vi "Recursive Folder List2.vi"(4 "Folders to Exclude\nREP ( ^[_.] as Default)\nempty to disable this feature":string="^[_.]", 6 "pattern":string, 8 "error in (no error)":errorcluster, 9 "Continue Recursing on Error? (F)":bool, 11 "Folder Path":path) -> (0 "error out":errorcluster, 1 "Number of Folders":i32, 2 "All Folders":path[](array[path]), 3 "dup Folder Path":path)   [LabVIEW 2017]
doc: "Recursively lists every folder under Folder Path whose name matches pattern. Folders to Exclude takes a regular expression and defaults to ^[_.], so hidden and underscore-prefixed folders are skipped."
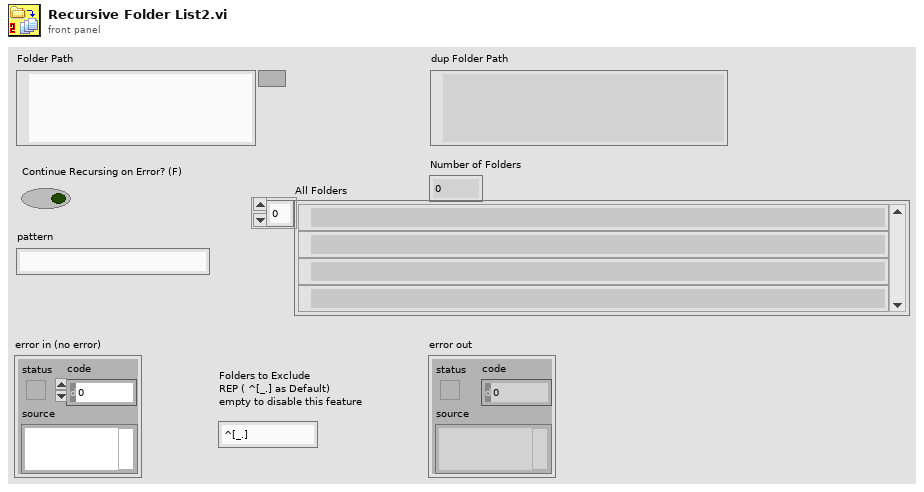
[diagram p1: front panel]
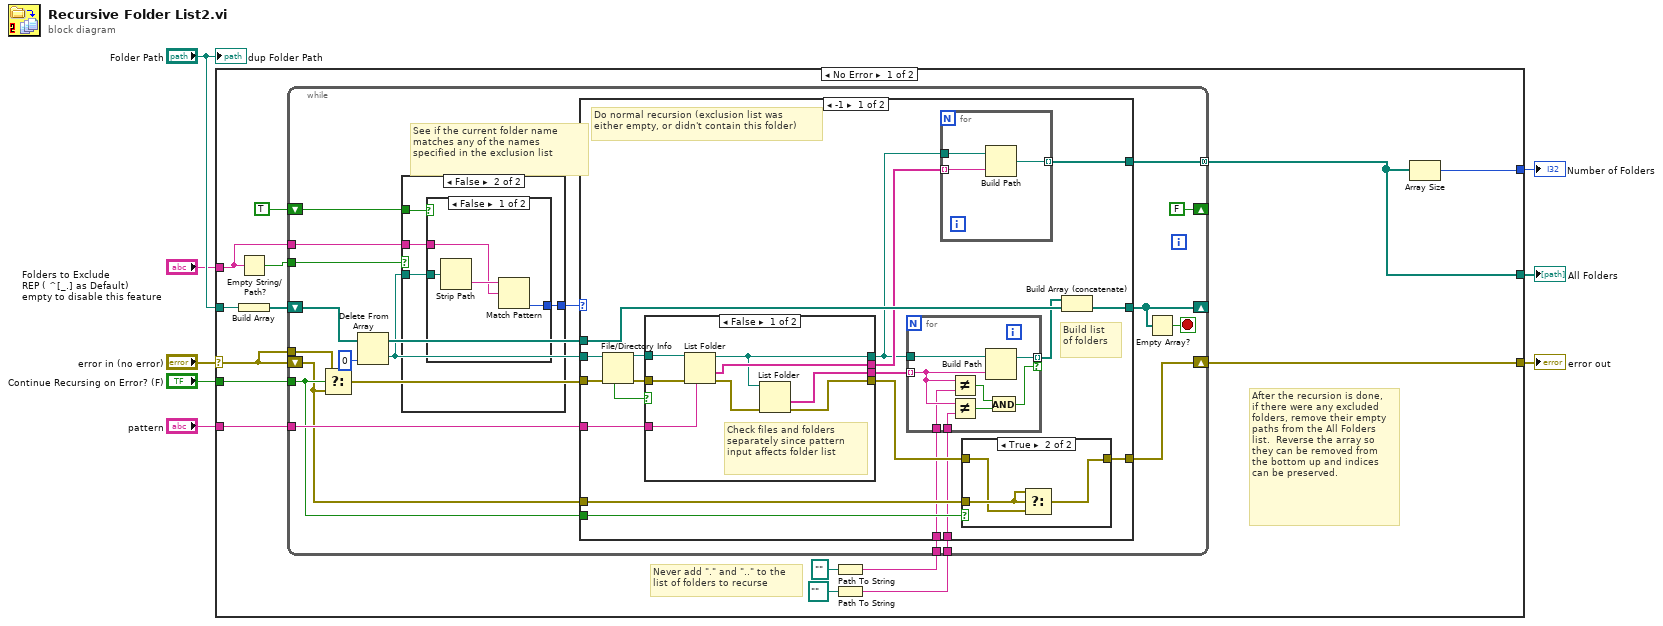
[diagram p0: block diagram]
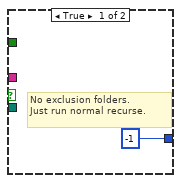
[diagram p2: hidden frame]
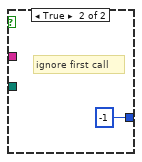
[diagram p3: hidden frame]
diagram:
  n1 = case shown="No Error" "error in (no error)" {
    selector: "error in (no error)" -> [w17 w100]
    tunnel: "Folder Path" -> [w23 _]
    tunnel: [w19 _] -> w8
    tunnel: [w20 w100] -> w7
    tunnel: [w9 _] -> w5
    tunnel: "pattern" -> [w21 _]
    tunnel: "Continue Recursing on Error? (F)" -> [w18 _]
    tunnel: "Folders to Exclude\nREP ( ^[_.] as Default)\nempty to disable this feature" -> [w11 _]
    frame No Error {
      # "Never add \".\" and \"..\" to the list of folders to recurse"
      # "After the recursion is done,\nif there were any excluded\nfolders, remove their empty\npaths from the All Folders\nlist.  Reverse the array so\nthey can be removed from\nthe bottom up and indices\ncan be preserved."
      n2 = Empty String/Path?(string/path=w11) -> (empty?=w12:bool)
      n3 = Build Array(w23) -> (w22:path[])
      n4 = Path To String(path=path "") -> (string=w14:string)
      n5 = Path To String(path=path "..") -> (string=w13:string)
      n6 = while {
        shift-left: w22 -> [w43]
        shift-right: [w41] -> _
        shift-right: [w35] -> w20
        shift-left: w17 -> [w34]
        tunnel: w21 -> [w42]
        tunnel: w18 -> [w36]
        tunnel: w17 -> [w37]
        tunnel: w11 -> [w31]
        tunnel: w12 -> [w32]
        tunnel: w14 -> [w28]
        tunnel: w13 -> [w27]
        shift-right: [FALSE] -> _
        shift-left: TRUE -> [w26]
        tunnel: [w24] -> w9 mode=concatenating
        stop <- w40 stop-if-true
        # "See if the current folder name\nmatches any of the names\nspecified in the exclusion list"
        n7 = Select(t=w37, s=w36, f=w34) -> (s? t:f=w38:errorcluster)
        n8 = Delete From Array(array=w43, index=0) -> (deleted portion=w30:path, array with subset deleted=w33:path[])  [unwired: 1 in]
        n9 = case shown="False" w32 {
          tunnel: w31 -> [_ w47]
          tunnel: w30 -> [_ w48]
          tunnel: [-1 ("index of element") w46] -> w29
          tunnel: w26 -> [_ w45]
          frame True {
            # "No exclusion folders.\nJust run normal recurse."
          }
          frame False {
            n10 = case shown="False" w45 {
              tunnel: w48 -> [w52 _]
              tunnel: w47 -> [w50 _]
              tunnel: [w49 -1 ("offset past match")] -> w46
              frame False {
                n11 = Strip Path(path=w52) -> (name=w51:string)  [unwired: 1 out]
                n12 = Match Pattern(string=w51, regular expression=w50) -> (offset past match=w49:i32)  [unwired: 1 in, 3 out]
              }
              frame True {
                # "ignore first call"
              }
            }
          }
        }
        n13 = case shown="-1" w29 {
          tunnel: w42 -> [w72 _]
          tunnel: [w70 w99] -> w41
          tunnel: w30 -> [w60 _]
          tunnel: w38 -> [w66 w98]
          tunnel: w36 -> [w64 _]
          tunnel: [w63 w98] -> w35
          tunnel: w34 -> [w62 _]
          tunnel: w33 -> [w61 w99]
          tunnel: w28 -> [w58 _]
          tunnel: w27 -> [w57 _]
          tunnel: [w54 _] -> w24
          frame -1 {
            # "Build list\nof folders"
            # "Do normal recursion (exclusion list was\neither empty, or didn't contain this folder)"
            n14 = File/Directory Info(path=w60, error in=w66) -> (path out=w68:path, error out=w69:errorcluster, shortcut=w67:bool)  [unwired: 4 out]
            n15 = case shown="False" w67 {
              tunnel: [w91 _] -> w56
              tunnel: [w90 w93] -> w55
              tunnel: [w89 w92] -> w65
              tunnel: w72 -> [w88 _]
              tunnel: [w84 _] -> w71
              tunnel: w69 -> [w87 w92]
              tunnel: w68 -> [w86 w93]
              frame False {
                # "Check files and folders\nseparately since pattern\ninput affects folder list"
                n16 = List Folder(path=w86, pattern=w88, error in=w87) -> (path out=w90:path, folder names=w91:string[], error out=w85:errorcluster)  [unwired: 2 out]
                n17 = List Folder(path=w90, error in=w85) -> (folder names=w84:string[], error out=w89:errorcluster)  [unwired: 4 out]
              }
              frame True {
                # "Do not attempt to recurse the contents of folder shortcuts"
              }
            }
            n18 = for {
              tunnel: w55 -> [w83]
              tunnel: [w82] -> w59 mode=indexing if=w81
              tunnel: w71 -> [w80] mode=indexing
              tunnel: w58 -> [w79]
              tunnel: w57 -> [w78]
              n19 = Not Equal?(x=w80, y=w79) -> (x != y?=w76:bool)
              n20 = Not Equal?(x=w80, y=w78) -> (x != y?=w77:bool)
              n21 = Build Path(base path=w83, name or relative path=w80) -> (appended path=w82:path)
              n22 = And(x=w76, y=w77) -> (x .and. y?=w81:bool)
            }
            n23 = for {
              tunnel: w56 -> [w75] mode=indexing
              tunnel: w55 -> [w74]
              tunnel: [w73] -> w54 mode=indexing
              n24 = Build Path(base path=w74, name or relative path=w75) -> (appended path=w73:path)
            }
            n25 = case shown="True" w64 {
              tunnel: w65 -> [w94 w96]
              tunnel: [w94 w95] -> w63
              tunnel: w62 -> [_ w97]
              frame False {
              }
              frame True {
                n26 = Select(t=w97, s=w97, f=w96) -> (s? t:f=w95:errorcluster)
              }
            }
            n27 = Build Array (concatenate)(w59, w61) -> (w70:path[])
          }
          frame Default {
            # "Output empty folder path here"
          }
        }
        n28 = Empty Array?(array=w41) -> (empty?=w40:bool)
      }
      n29 = Array Size(array=w9) -> (size(s)=w19:i32)
    }
    frame Error {
    }
  }
  "Number of Folders" <- w8
  "error out" <- w7
  "All Folders" <- w5
  "dup Folder Path" <- "Folder Path"
